vi "Read Waveform.vi"(0 "VISA resource name":refnum<visa-resource-name>, 5 "Channel (1)":i32(ring)=1 items=["1"=1, "2"=2, "3"=3, "4"=4], 9 "Maximum Time (5000)":i32=5000, 11 "error in (no error)":errorcluster) -> (4 "VISA resource name out":refnum<visa-resource-name>, 6 "Waveform Array":dbl[](array[numeric]) format="%^.3e", 8 "Actual Points":i32, 10 "Initial X":dbl format="%^.3e", 14 "X Increment":dbl format="%^.3e", 15 "error out":errorcluster)   [LabVIEW 2020, in "Rohde&Schwarz RTx Oscilloscopes.lvlib"]
doc: "This VI initiates an acquisition on the channels that you enable with the Configure Channel.vi. It then waits for the acquisition to complete, and returns the waveform for the channel you specify. You call the Fetch Waveform.vi to obtain the waveforms for each of the remaining enabled channels without initiating another acquisition.\n\nNotes:\n- After this VI executes, each element in the Waveform Array parameter is either a voltage or a value indicating that the oscilloscope could not sample a voltage.\n- You configure the interpolation method the oscilloscope uses with the Configure Interpolation.vi. If you disable interpolation, the oscilloscope does not interpolate points in the waveform.\n\nAttributes:\nRSRTX_ATTR_RUN_SINGLE_WAIT_FOR_OPC\nRSRTX_ATTR_WAVEFORM_CONVERSION_X_START\nRSRTX_ATTR_WAVEFORM_CONVERSION_X_INCREMENT\n\nRemote-control commands:\nSINGle\nCHANnel<m>:DATA:XORigin?\nCHANnel<m>:DATA:XINCrement?\nFORMat[:DATA]\nCHANnel<m>:DATA?"
uses:
  Rohde&Schwarz RTx Oscilloscopes.lvlib
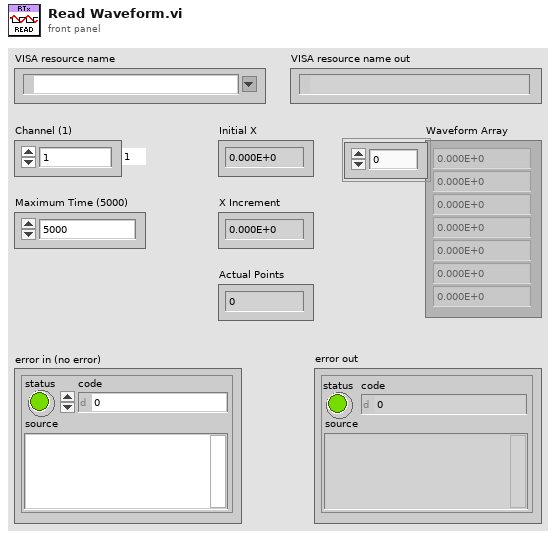
[diagram p1: front panel]
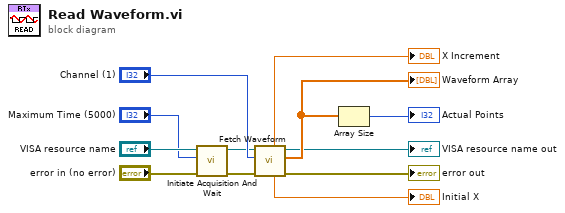
[diagram p0: block diagram]
diagram:
  n1 = call "Initiate Acquisition And Wait.vi"("error in (no error)"="error in (no error)", "Maximum Time (5000)"="Maximum Time (5000)", "VISA resource name"="VISA resource name") -> ("error out"=w5:errorcluster, "VISA resource name out"=w4:refnum<visa-resource-name>)  [unwired: 7 in]
  n2 = call "Fetch Waveform.vi"("error in (no error)"=w5, "Channel (1)"="Channel (1)", "VISA resource name"=w4) -> ("error out"=→"error out":errorcluster, "Waveform Array"=w10:dbl[], "VISA resource name out"=→"VISA resource name out":refnum<visa-resource-name>, "Initial X"=→"Initial X":dbl, "X Increment"=→"X Increment":dbl)  [unwired: 4 in]
  "Waveform Array" <- w10
  n3 = Array Size(array=w10) -> (size(s)=→"Actual Points":i32)
